vi "ex01_d.vi"() -> ()   [LabVIEW 2011]
panel:
  out "String 4":string
  out "String 3":string
  in  "stop":bool
  out "String 2":string
  in  "String":string
  out "Boolean 3":bool
  in  "OK Button":bool
  in  "Boolean 2":bool
  in  "Numeric Control":dbl
  out "Boolean":bool
  out "Gauge":dbl(knob) scale=0.0..10.0
  in  "Knob":dbl(knob) scale=0.0..10.0
  in  "Numeric":dbl
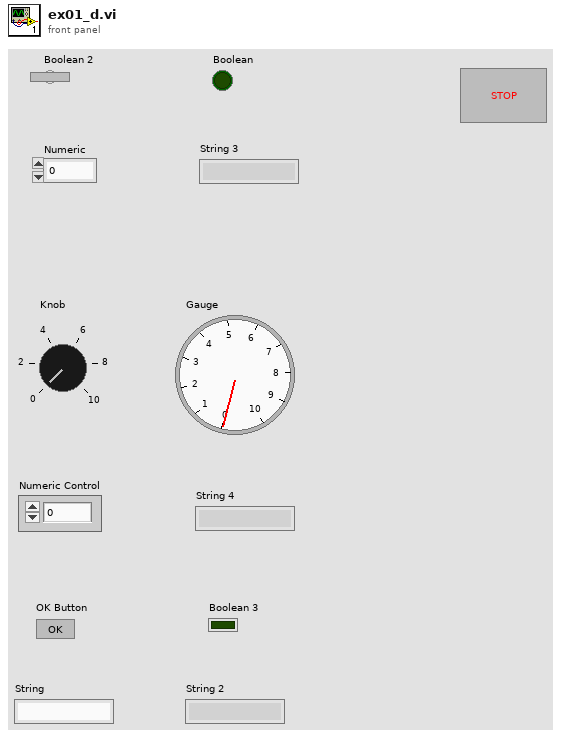
[diagram p1: front panel]
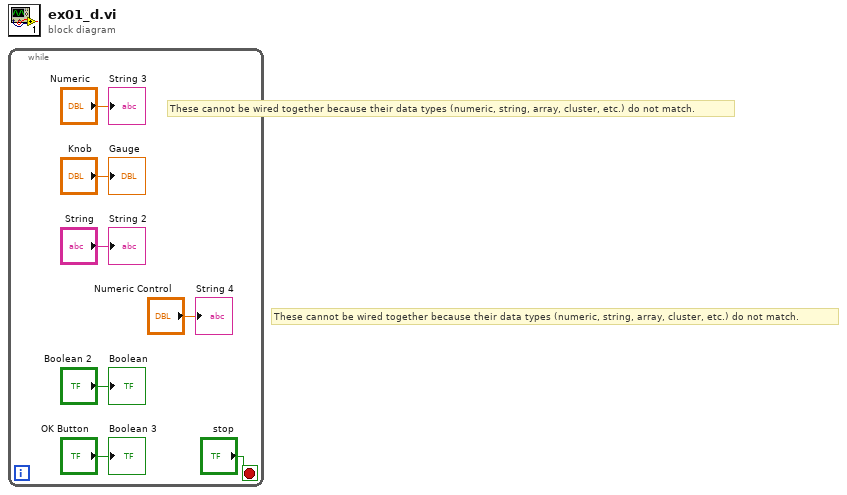
[diagram p0: block diagram]
diagram:
  # "These cannot be wired together because their data types (numeric, string, array, cluster, etc.) do not match."
  # "These cannot be wired together because their data types (numeric, string, array, cluster, etc.) do not match."
  n1 = while {
    stop <- "stop" stop-if-true
    "Gauge" <- "Knob"
    "Boolean" <- "Boolean 2"
    "Boolean 3" <- "OK Button"
    "String 2" <- "String"
    "String 3" <- "Numeric"
    "String 4" <- "Numeric Control"
  }
